vi "均值.vi"() -> ()   [LabVIEW 2018]
uses:
  <vilib>/gmath/NI_Gmath.lvlib
panel:
  in  "停止":bool
  out "mean value":dbl caption="均值"
  in  "percent (trim)":dbl=25.0 caption="百分比(取整)"
  in  "type":T1(ring) caption="类型"
  in  "数组":dbl[](array[numeric])
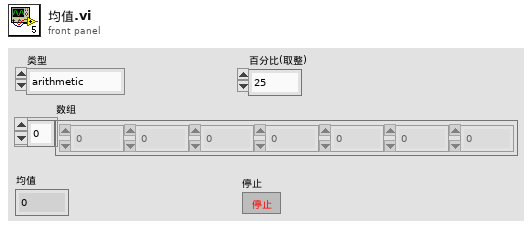
[diagram p1: front panel]
types:
  T1 = enum16{"arithmetic", "geometric", "harmonic", "trimmed", "median"}
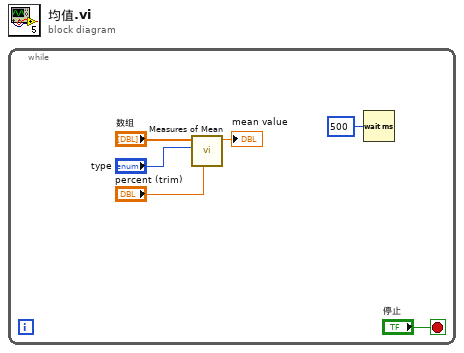
[diagram p0: block diagram]
diagram:
  n1 = while {
    stop <- "停止" stop-if-true
    n2 = call <vilib>:"Measures of Mean.vi"("percent (trim)"="percent (trim)", "type"="type", "x array"="数组") -> ("mean value"=→"mean value":dbl)  [unwired: 7 in, 1 out]
    n3 = Wait (ms)(milliseconds to wait=u32 500 ("等待时间（毫秒）")) -> ()  [unwired: 1 out]
  }
